vi "TrapTest-2017-06-06.vi"() -> ()   [LabVIEW 2010]
uses:
  <vilib>/userDefined/High Color/nirio_resource_hc.ctl
  <vilib>/rvi/interface/nirviOpenFPGA/nirviOpenFPGA.xnode
  C:/Users/HAGAR-IV/Desktop/Zeugs/markus/version feb 2012/FPGA Bitfiles/pertrasgcfpga2_FPGATarget_Trap1-06-06-2017_7789B2A8.lvbitx
  C:/Users/HAGAR-IV/Desktop/Zeugs/Johnny/pertrasgc fpga/Trap1-06-06-2017.vi
  <vilib>/rvi/ClientSDK/nirviWhatTheDeviceIsDoing.ctl
  <vilib>/rvi/interface/nirviReadWriteControl/nirviReadWriteControl.xnode
  <vilib>/rvi/interface/common/niFpgaNodeNameForErrorReporting.ctl
  <vilib>/rvi/errors/niLvFpgaWhatHappensToTopLevelVI.ctl
  <vilib>/rvi/interface/nirviMethod/nirviMethod.xnode
  <vilib>/rvi/interface/nirviCloseFPGA/nirviCloseFPGA.xnode
  <vilib>/FPGAPlugInAG/cRIO-9114/niLvFpga_Open_cRIO-9114.vi
  <vilib>/rvi/interface/common/dynamic/niFpgaDynamicAddResources.vi
  <vilib>/Utility/error.llb/Error Cluster From Error Code.vi
  <vilib>/rvi/errors/niLvFpgaAdjustHostInterfaceError.vi
  <vilib>/FPGAPlugInAG/Dynamic/niLvFpga_Close_Dynamic.vi
  NiFpgaLv.dll
panel:
  out "dT":dbl
  out "StirlingTemp":dbl
  out "Heizrate":dbl[](graph)
  in  "Stirling":bool
  in  "d1_Regelung":fxp<+/-,21,21>
  in  "d0_Regelung":fxp<+/-,18,18>
  out "U_SP":dbl
  in  "tau":dbl
  out "U_MW":dbl
  out "R":dbl
  out "T":dbl
  in  "heizen":bool
  in  "Löschen":bool
  out "TheWireTemp":dbl[](graph)
  in  "stop":bool
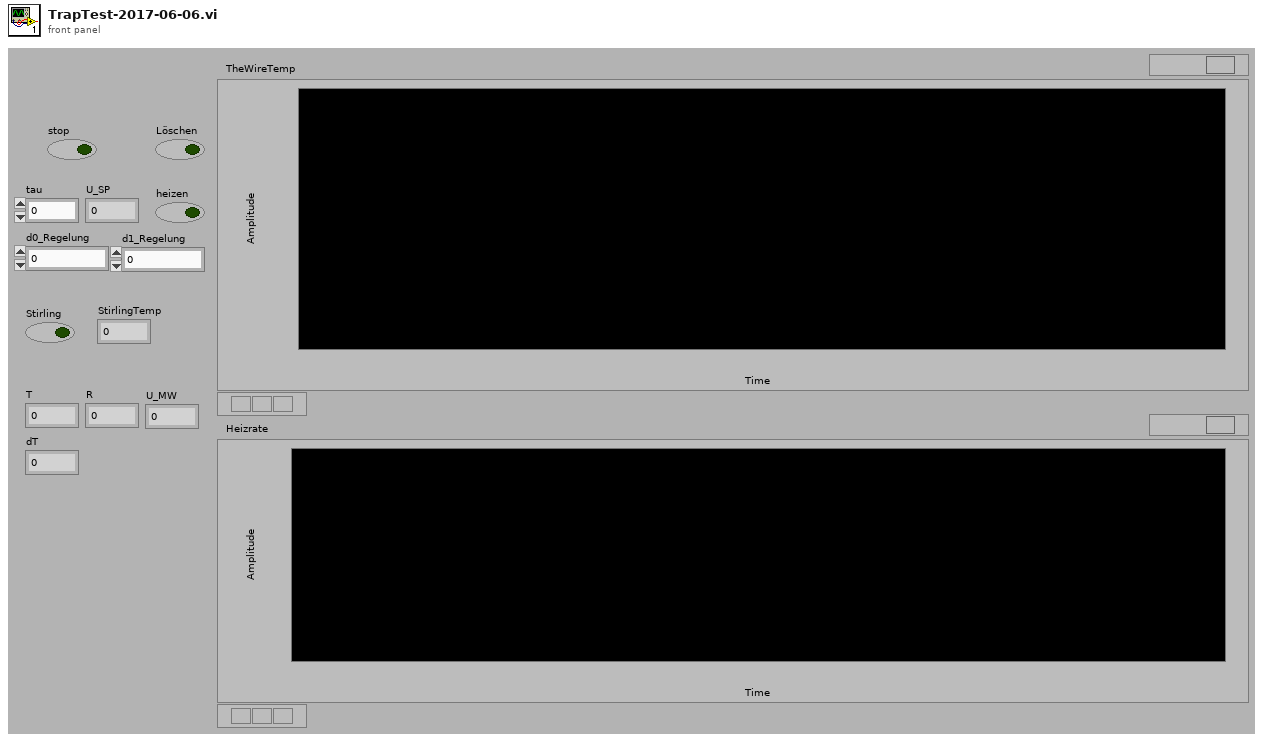
[diagram p1: front panel]
types:
  T1 = typedef "niFpgaNodeNameForErrorReporting.ctl" = enum16{"Open FPGA VI Reference", "Read/Write Control", "Invoke Method: Abort", "Invoke Method: Acknowledge IRQ", "Invoke Method: Download", "Invoke Method: FIFO.Configure", "Invoke Method: FIFO.Read", "Invoke Method: FIFO.Start", "Invoke Method: FIFO.Stop", "Invoke Method: FIFO.Write", "Invoke Method: Reset", "Invoke Method: Run", "Invoke Method: Wait on IRQ", "Close FPGA VI Reference"}
  T2 = typedef "niLvFpgaWhatHappensToTopLevelVI.ctl" = enum16{"top level VI scripted behind XNode", "top level VI inlined behind XNode"}
  T3 = typedef "nirviWhatTheDeviceIsDoing.ctl" = enum32{"nothing", "something other than LabVIEW FPGA", "FPGA interface", "interactive", "emulation"}
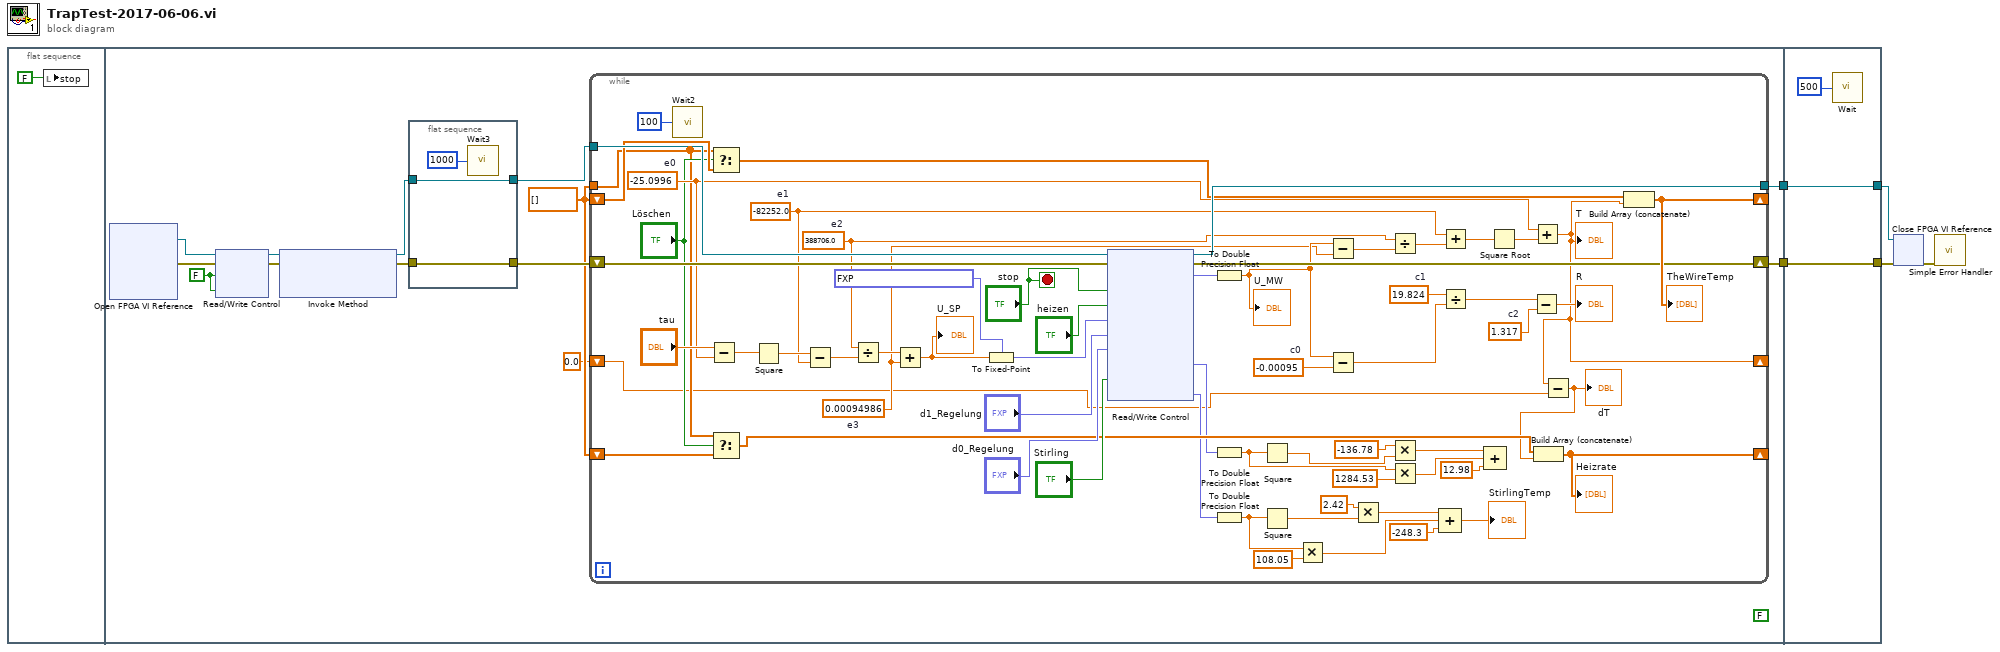
[diagram p0: block diagram]
diagram:
  n1 = flat-sequence {
    tunnel: [w15] -> w5
    tunnel: [w14] -> w3
    tunnel: w5 -> [w508]
    tunnel: [w508] -> w4
    tunnel: w3 -> [w507]
    tunnel: [w507] -> w2
    frame #0 {
      n2 = local write "stop"(FALSE ("stop")) -> ()
    }
    frame #1 {
      (unwired) FALSE
      w8 = dbl[] []
      w13 = FALSE ("stop")
      n3 = xnode "Open FPGA VI Reference"() -> ("FPGA VI Reference Out"=w19:refnum<k20>, "error out"=w18:errorcluster)  [unwired: 2 in]
      n4 = xnode "Read/Write Control"("FPGA VI Reference In"=w19, "error in"=w18, "stop"=w13, "heizen"=w13) -> ("FPGA VI Reference Out"=w17:refnum<k20>, "error out"=w16:errorcluster)
      n5 = xnode "Invoke Method"("FPGA VI Reference In"=w17, "error in"=w16) -> ("FPGA VI Reference Out"=w12:refnum<k20>, "error out"=w10:errorcluster)  [unwired: 1 in]
      n6 = flat-sequence {
        tunnel: w12 -> [w22]
        tunnel: [w22] -> w11
        tunnel: w10 -> [w21]
        tunnel: [w21] -> w9
        frame #0 {
          n7 = call "Wait3"("Count(mSec)"=u32 1000) -> ()  [unwired: 1 out]
        }
      }
      n8 = while {
        tunnel: w11 -> [w84]
        shift-right: [w82] -> _
        shift-left: w8 -> [w78]
        tunnel: [w81] -> w15
        shift-right: [w80] -> w14
        shift-left: w9 -> [w83]
        tunnel: w8 -> [w47]
        shift-right: [w44] -> _
        shift-left: w8 -> [w46]
        shift-right: [w25] -> _
        shift-left: 0.0 -> [w24]
        stop <- "stop" stop-if-true
        w64 = 1.317  # c2
        w67 = 19.824  # c1
        w68 = -0.00095  # c0
        w54 = 0.00094986  # e3
        w57 = 388706.0  # e2
        w58 = -82252.0  # e1
        w61 = -25.0996  # e0
        n9 = call "Wait2"("Count(mSec)"=u32 100) -> ()  [unwired: 1 out]
        n10 = Subtract(x="tau", y=w61) -> (x-y=w60:dbl)
        n11 = Select(t=w47, s="Löschen", f=w78) -> (s? t:f=w77:dbl[])
        n12 = Select(t=w47, s="Löschen", f=w46) -> (s? t:f=w45:dbl[])
        n13 = Square(x=w60) -> (x^2=w59:dbl)
        n14 = Subtract(x=w59, y=w58) -> (x-y=w56:dbl)
        n15 = Divide(x=w57, y=w56) -> (x/y=w55:dbl)
        n16 = Add(x=w55, y=w54) -> (x+y=w53:dbl)
        "U_SP" <- w53
        n17 = To Fixed-Point(fixed-point type=fxp<+/-,26,5> 0.0, number=w53) -> (fixed-point=w51:fxp<+/-,26,5>)
        n18 = xnode "Read/Write Control"("FPGA VI Reference In"=w84, "error in"=w83, "stop"="stop", "heizen"="heizen", "U_SP"=w51, "d1"="d1_Regelung", "d0"="d0_Regelung", "Stirling"="Stirling") -> ("FPGA VI Reference Out"=w81:refnum<k20>, "error out"=w80:errorcluster, "U_MW"=w74:fxp<+/-,26,5>, "PreCol1_MW"=w43:fxp<+/-,26,5>, "PTStirling"=w28:fxp<+/-,26,5>)
        n19 = To Double Precision Float(number=w74) -> (double precision float=w69:dbl)
        "U_MW" <- w69
        n20 = To Double Precision Float(number=w43) -> (double precision float=w41:dbl)
        n21 = To Double Precision Float(number=w28) -> (double precision float=w34:dbl)
        n22 = Square(x=w41) -> (x^2=w40:dbl)
        n23 = Square(x=w34) -> (x^2=w33:dbl)
        n24 = Multiply(x=w34, y=108.05) -> (x*y=w30:dbl)
        n25 = Subtract(x=w69, y=w54) -> (x-y=w73:dbl)
        n26 = Subtract(x=w69, y=w68) -> (x-y=w66:dbl)
        n27 = Multiply(x=2.42, y=w33) -> (x*y=w31:dbl)
        n28 = Divide(x=w57, y=w73) -> (x/y=w72:dbl)
        n29 = Multiply(x=-136.78, y=w40) -> (x*y=w38:dbl)
        n30 = Multiply(x=w41, y=1284.53) -> (x*y=w37:dbl)
        n31 = Compound Arithmetic op=ADD(w31, w30, -248.3 ("value")) -> (→"StirlingTemp":dbl)
        n32 = Add(x=w58, y=w72) -> (x+y=w71:dbl)
        n33 = Divide(x=w67, y=w66) -> (x/y=w65:dbl)
        n34 = Compound Arithmetic op=ADD(w38, w37, 12.98 ("value")) -> ()  [unwired: 1 out]
        n35 = Square Root(x=w71) -> (sqrt(x)=w70:dbl)
        n36 = Subtract(x=w65, y=w64) -> (x-y=→"R":dbl)
        n37 = Add(x=w61, y=w70) -> (x+y=w25:dbl)
        "T" <- w25
        n38 = Subtract(x=w25, y=w24) -> (x-y=w23:dbl)
        "dT" <- w23
        n39 = Build Array (concatenate)(w45, w23) -> (w44:dbl[])
        "Heizrate" <- w44
        n40 = Build Array (concatenate)(w77, w25) -> (w82:dbl[])
        "TheWireTemp" <- w82
      }
    }
    frame #2 {
      n41 = call "Wait"("Count(mSec)"=u32 500) -> ()  [unwired: 1 out]
    }
  }
  n42 = xnode "Close FPGA VI Reference"("FPGA VI Reference In"=w4, "error in"=w2) -> ("error out"=w1:errorcluster)
  n43 = call <vilib>:"Simple Error Handler.vi"("error in (no error)"=w1) -> ()  [unwired: 4 in, 5 out]
